vi "Substitute Actor.vi"(10 "Substitute Actor in":refnum<class "Actor.lvclass">, 11 "Current Actor":refnum<class "Actor.lvclass">) -> (0 "error out":errorcluster, 2 "Substitute Actor out":refnum<class "Actor.lvclass">)   [LabVIEW 2020, in "Actor Framework.lvlib" / "Actor.lvclass"]
doc: "(<B>Filename</B>: Actor Framework.lvlib:Actor.lvclass:Substitute Actor.vi)\n\nThis method copies information from the <b>Current Actor</b> to the <b>Substitute Actor</b>, including the to-self and the to-caller queue references. The purpose of this function is to allow an actor to define a method that replaces itself with another actor, useful for implementing a State Pattern Actor. Child classes should override this method to copy any additional fields that they need from the current to the substitute.\n\nThis method may return error code 678010: Illegal substitution. Overrides of this method may choose to return this error if the new actor is not one that is an appropriate substitute for the current actor, for whatever standards of \"appropriate\" are chosen for the current actor. If returning an error, override VIs should return the unmodified <b>Current Actor</b> as <b>Substitute Actor out</b>."
uses:
  Actor.lvclass
  Actor.lvclass/Actor.ctl
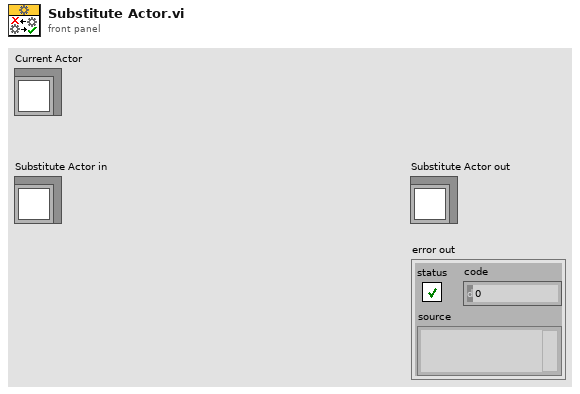
[diagram p1: front panel]
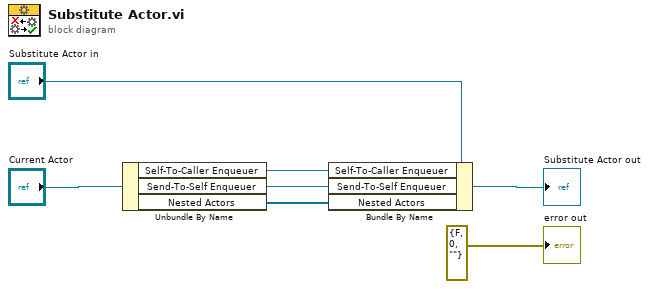
[diagram p0: block diagram]
diagram:
  n1 = Unbundle By Name("Current Actor") -> ("Self-To-Caller Enqueuer"=w5:refnum<class "Message Enqueuer.lvclass">, "Send-To-Self Enqueuer"=w4:refnum<class "Message Priority Queue.lvclass">, "Nested Actors"=w1:refnum<class "Message Enqueuer.lvclass">[])
  n2 = Bundle By Name(cluster="Substitute Actor in", "Self-To-Caller Enqueuer"=w5, "Send-To-Self Enqueuer"=w4, "Nested Actors"=w1) -> (→"Substitute Actor out":refnum<class "Actor.lvclass">)
  "error out" <- errorcluster {"status"=FALSE, "code"=0, "source"=""} ("error out")
